vi "subXMLGetItemURLFromReferencePath.vi"(9 "Reference path":string, 11 "Root ref":refnum<k20>) -> (1 "Path":path, 2 "Found?":bool, 3 "Refnum out":refnum<k20>)   [LabVIEW 2019, in "SolutionBuilder.lvlib" / "SolutionBuilder.lvclass"]
uses:
  SolutionBuilder.lvclass
  <vilib>/regexp/Match Regular Expression.xnode
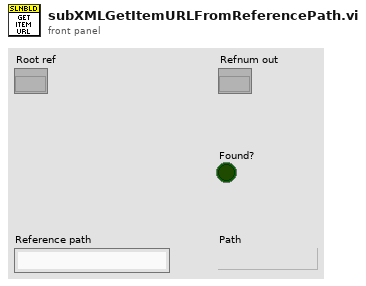
[diagram p1: front panel]
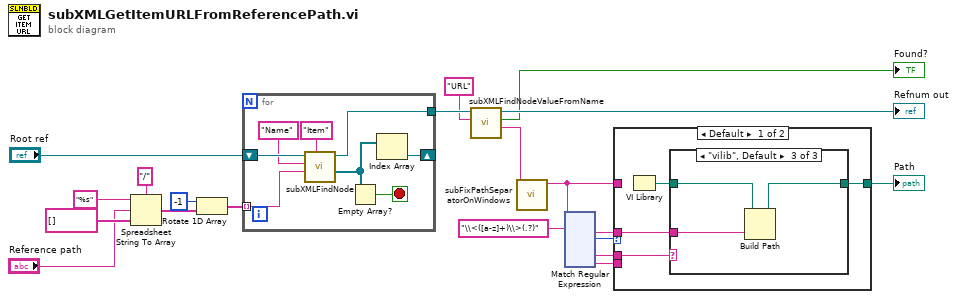
[diagram p0: block diagram]
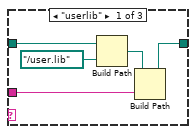
[diagram p2: hidden frame]
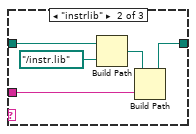
[diagram p3: hidden frame]
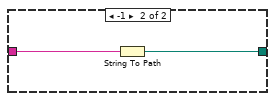
[diagram p4: hidden frame]
diagram:
  n1 = Spreadsheet String To Array(delimiter (Tab)="/", format string="%s", spreadsheet string="Reference path", array type (2D Dbl)=string[] [] ("Names")) -> (array=w12:string[])
  n2 = Rotate 1D Array(1:w12, 2:-1 ("n")) -> (0:w10:string[])
  n3 = for {
    shift-right: [w23] -> _
    shift-left: "Root ref" -> [w28]
    tunnel: w10 -> [w27] mode=indexing
    tunnel: [w21] -> w15
    stop <- w22 stop-if-true
    n4 = call "subXMLFindNode.vi"("Node name"="Item", "Property value"=w27, "Property name"="Name", "Refnum in"=w28) -> ("Nodes"=w24:refnum<k20>[], "Refnum"=w21:refnum<k20>)  [unwired: 6 in]
    n5 = Empty Array?(array=w24) -> (empty?=w22:bool)
    n6 = Index Array(array=w24) -> (element=w23:refnum<k20>)  [unwired: 1 in]
  }
  n7 = call "subXMLFindNodeValueFromName.vi"("Property name"="URL", "Refnum in"=w15) -> ("Value"=w2:string, "Found?"=→"Found?":bool, "Refnum out"=→"Refnum out":refnum<k20>)  [unwired: 7 in]
  n8 = call "subFixPathSeparatorOnWindows.vi"("Value"=w2) -> ("fixed path"=w1:string)  [unwired: 10 in]
  n9 = xnode "Match Regular Expression"("input string"=w1, "regular expression"="\\<([a-z]+)\\>(.?)") -> ("after match"=w4:string, "offset past match"=w5:i32, "submatch 1"=w6:string, "submatch 2"=w3:string)  [unwired: 4 in, 3 out]
  n10 = case shown="Default" w5 {
    tunnel: [w30 w47] -> w9
    tunnel: w1 -> [_ w46]
    tunnel: w6 -> [w32 _]
    tunnel: w4 -> [w29 _]
    tunnel: w3 -> [_ _]
    frame Default {
      n11 = VI Library() -> (path=w31:path)
      n12 = case shown="\"vilib\", Default" w32 {
        tunnel: w31 -> [w37 w42 w45]
        tunnel: [w33 w38 w44] -> w30
        tunnel: w29 -> [w34 w39 w43]
        frame "userlib" {
          n13 = Build Path(base path=w37, name or relative path=path "../user.lib" ("path")) -> (appended path=w35:path)
          n14 = Build Path(base path=w35, name or relative path=w34) -> (appended path=w33:path)
        }
        frame "instrlib" {
          n15 = Build Path(base path=w42, name or relative path=path "../instr.lib" ("path")) -> (appended path=w40:path)
          n16 = Build Path(base path=w40, name or relative path=w39) -> (appended path=w38:path)
        }
        frame "vilib", Default {
          n17 = Build Path(base path=w45, name or relative path=w43) -> (appended path=w44:path)
        }
      }
    }
    frame -1 {
      n18 = String To Path(string=w46) -> (path=w47:path)
    }
  }
  "Path" <- w9
